vi "BoxMuellerAlgorithmSubVI.vi"() -> (0 "Uniform Deviate 2":dbl, 1 "Uniform Deviate 1":dbl, 2 "g":dbl, 3 "s":dbl)   [LabVIEW 2019]
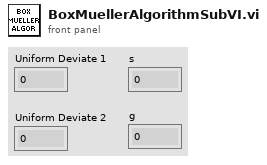
[diagram p1: front panel]
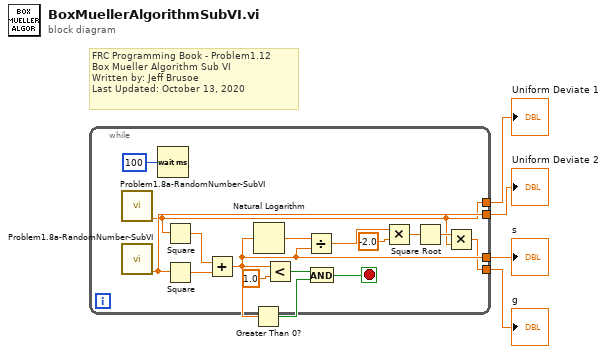
[diagram p0: block diagram]
diagram:
  # "FRC Programming Book - Problem1.12\nBox Mueller Algorithm Sub VI\nWritten by: Jeff Brusoe\nLast Updated: October 13, 2020"
  n1 = while {
    tunnel: [w8] -> w1
    tunnel: [w7] -> w2
    tunnel: [w5] -> w3
    tunnel: [w6] -> w4
    stop <- w20 stop-if-true
    n2 = call "Problem1.8a-RandomNumber-SubVI.vi"() -> ("Uniform Deviate"=w5:dbl)  [unwired: 10 in, 1 out]
    n3 = call "Problem1.8a-RandomNumber-SubVI.vi"() -> ("Uniform Deviate"=w6:dbl)  [unwired: 10 in, 1 out]
    n4 = Wait (ms)(milliseconds to wait=u32 100) -> ()  [unwired: 1 out]
    n5 = Square(x=w5) -> (x^2=w16:dbl)
    n6 = Square(x=w6) -> (x^2=w15:dbl)
    n7 = Add(x=w16, y=w15) -> (x+y=w8:dbl)
    n8 = Greater Than 0?(x=w8) -> (x > 0?=w19:bool)
    n9 = Natural Logarithm(1:w8) -> (0:w13:dbl)
    n10 = Less?(x=w8, y=1.0) -> (x < y?=w18:bool)
    n11 = Divide(x=w13, y=w8) -> (x/y=w12:dbl)
    n12 = And(x=w18, y=w19) -> (x .and. y?=w20:bool)
    n13 = Multiply(x=w12, y=-2.0) -> (x*y=w10:dbl)
    n14 = Square Root(x=w10) -> (sqrt(x)=w9:dbl)
    n15 = Multiply(x=w9, y=w5) -> (x*y=w7:dbl)
  }
  "g" <- w2
  "s" <- w1
  "Uniform Deviate 2" <- w4
  "Uniform Deviate 1" <- w3
